vi "WPI_DigitalOutputGeneratePWM.vi"(8 "error in (no error)":errorcluster, 10 "PWM Duty Cycle":sgl, 11 "DigitalOutputDevRef":T1={"DIO Channel"=enum."DIO 1", "DevStatus"={"status"=FALSE, "code"=0, "source"=""}}) -> (0 "error out":errorcluster, 3 "DigitalOutputDevRef":T1={"DIO Channel"=enum."DIO 1", "DevStatus"={"status"=FALSE, "code"=0, "source"=""}})   [LabVIEW 2017]
doc: "Generates a PWM signal on a Digital Output channel.\n\nThe resolution of the duty cycle is 8-bit for low frequencies (1kHz or less) but is reduced the higher the frequency of the PWM signal is.\n\nThis software is licensed. Open the labview\\readme\\WPI Robotics Library Open Source License.txt file for more information."
uses:
  <vilib>/Rock Robotics/WPI/DigitalOutput/WPI_DigitalOutputDevRef.ctl
  <vilib>/Rock Robotics/SystemInterfaces/DIO/FPGA_DIOChannel.ctl
  <vilib>/Rock Robotics/WPI/DigitalModule/WPI_DigitalModuleDIOCacheOp.ctl
  <vilib>/Rock Robotics/SystemInterfaces/System/FPGA_SystemGet.vi
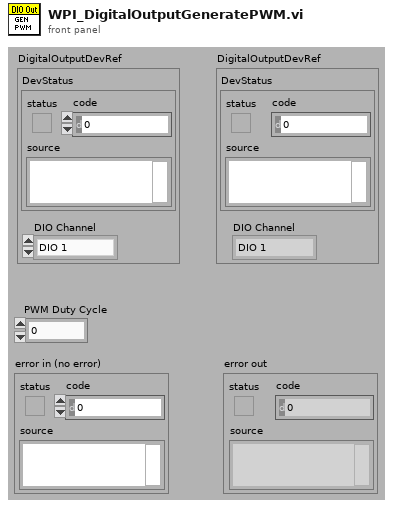
[diagram p1: front panel]
types:
  T1 = typedef "WPI_DigitalOutputDevRef.ctl" = cluster{"DIO Channel":T2, "DevStatus":errorcluster}
  T2 = typedef "FPGA_DIOChannel.ctl" = enum8{"DIO 0", "DIO 1", "DIO 2", "DIO 3", "DIO 4", "DIO 5", "DIO 6", "DIO 7", "DIO 8", "DIO 9", "DIO MXP 0", "DIO MXP 1", "DIO MXP 2", "DIO MXP 3", "DIO MXP 4", "DIO MXP 5", "DIO MXP 6", "DIO MXP 7", "DIO MXP 8", "DIO MXP 9", "DIO MXP 10", "DIO MXP 11", "DIO MXP 12", "DIO MXP 13", "DIO MXP 14", "DIO MXP 15", "SPI Port CS1", "SPI Port CS2", "SPI Port CS3", "SPI Port MISO", "SPI Port MOSI", "Invalid"}
  T3 = typedef "WPI_DigitalModuleDIOCacheOp.ctl" = enum16{"Acquire", "Release", "Status"}
  T4 = typedef "WPI_DigitalOutputPWMRef.ctl" = enum16{"DO PWM 0", "DO PWM 1", "DO PWM 2", "DO PWM 3", "DO PWM 4", "DO PWM 5", "Invalid"}
  T5 = typedef "FPGA_DIODevRef.ctl" = cluster{"DevStatus":errorcluster}
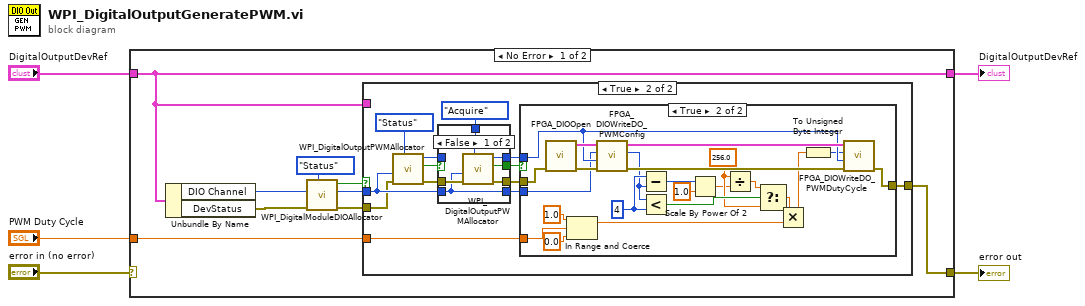
[diagram p0: block diagram]
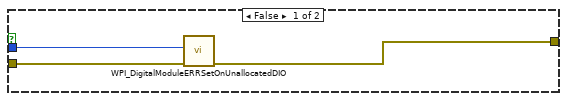
[diagram p2: hidden frame]
diagram:
  n1 = case shown="No Error" "error in (no error)" {
    selector: "error in (no error)" -> [_ w66]
    tunnel: "DigitalOutputDevRef" -> [w6 w65]
    tunnel: [w6 w65] -> w4
    tunnel: [w8 w66] -> w2
    tunnel: "PWM Duty Cycle" -> [w7 _]
    frame No Error {
      n2 = Unbundle By Name(w6) -> ("DIO Channel"=w13:T2, "DevStatus"=w12:errorcluster)
      n3 = call <vilib>:"WPI_DigitalModuleDIOAllocator.vi"("AllocatedDIOMutex"=WPI_DigitalModuleDIOCacheOp."Status", "error in (no error)"=w12, "DIOChannel"=w13) -> ("error out"=w9:errorcluster, "Allocated DIOChannel"=w11:T2, "AllocatedDIO"=w10:bool)  [unwired: 1 in, 5 out]
      n4 = case shown="True" w10 {
        tunnel: w7 -> [_ w18]
        tunnel: [w16 w19] -> w8
        tunnel: w11 -> [w15 w26]
        tunnel: w6 -> [_ _]
        tunnel: w9 -> [w17 w25]
        frame False {
          n5 = call <vilib>:"WPI_DigitalModuleERRSetOnUnallocatedDIO.vi"("error in (no error)"=w17, "DIOChannel"=w15) -> ("error out"=w16:errorcluster)  [unwired: 9 in]
        }
        frame True {
          n6 = call <vilib>:"WPI_DigitalOutputPWMAllocator.vi"("Operation"=WPI_DigitalModuleDIOCacheOp."Status", "error in (no error)"=w25, "DIO Channel"=w26) -> ("error out"=w24:errorcluster, "Allocated"=w29:bool, "PWM Allocated"=w28:T4)  [unwired: 2 in, 4 out]
          n7 = case shown="False" w29 {
            selector: w29 -> [_ w62]
            tunnel: w28 -> [_ w64]
            tunnel: [w60 w64] -> w22
            tunnel: WPI_DigitalModuleDIOCacheOp."Acquire" ("Operation") -> [w59 _]
            tunnel: w26 -> [w55 w61]
            tunnel: w24 -> [w58 w63]
            tunnel: [w57 w63] -> w20
            tunnel: [w56 w62] -> w23
            tunnel: [w55 w61] -> w21
            frame False {
              n8 = call <vilib>:"WPI_DigitalOutputPWMAllocator.vi"("Operation"=w59, "error in (no error)"=w58, "DIO Channel"=w55) -> ("error out"=w57:errorcluster, "Allocated"=w56:bool, "PWM Allocated"=w60:T4)  [unwired: 2 in, 4 out]
            }
            frame True {
            }
          }
          n9 = case shown="True" w23 {
            tunnel: w22 -> [_ w46]
            tunnel: w21 -> [_ w44]
            tunnel: w20 -> [w31 w51]
            tunnel: [w31 w47] -> w19
            tunnel: w18 -> [_ w43]
            frame False {
            }
            frame True {
              w38 = u8 4 ("y")
              w36 = 256.0 ("y")
              n10 = call <vilib>:"FPGA_DIOOpen.vi"("error in (no error)"=w51) -> ("error out"=w50:errorcluster, "DIODeviceRef"=w52:T5)  [unwired: 1 in, 8 out]
              n11 = In Range and Coerce(upper limit=1.0, x=w43, lower limit=0.0) -> (coerced(x)=w42:dbl)  [unwired: 1 out]
              n12 = call <vilib>:"FPGA_DIOWriteDO_PWMConfig.vi"("error in (no error)"=w50, "DO_PWM Index"=w46, "DO_PWMOutputSelect"=w44, "DIODeviceRef"=w52) -> ("error out"=w49:errorcluster, "DO_PWMPeriodPower Out"=w37:u16, "DIODeviceRef"=w48:T5)  [unwired: 1 in, 4 out]
              n13 = Subtract(x=w38, y=w37) -> (x-y=w33:u16)
              n14 = Less?(x=w37, y=w38) -> (x < y?=w40:bool)
              n15 = Scale By Power Of 2(n=w33, x=1.0) -> (x*2^n=w32:dbl)
              n16 = Divide(x=w36, y=w32) -> (x/y=w35:dbl)
              n17 = Select(t=w35, s=w40, f=w36) -> (s? t:f=w39:dbl)
              n18 = Multiply(x=w39, y=w42) -> (x*y=w41:dbl)
              n19 = To Unsigned Byte Integer(number=w41) -> (unsigned 8bit integer=w45:u8)
              n20 = call <vilib>:"FPGA_DIOWriteDO_PWMDutyCycle.vi"("error in (no error)"=w49, "DO_PWM Index"=w46, "DO_PWMDutyCycle"=w45, "DIODeviceRef"=w48) -> ("error out"=w47:errorcluster)  [unwired: 7 out]
            }
          }
        }
      }
    }
    frame Error {
    }
  }
  "DigitalOutputDevRef" <- w4
  "error out" <- w2
